vi "Obtain Broadcast Events.vi"(8 "error in (no error)":errorcluster, 10 "Create New? (F)":bool) -> (0 "error out":errorcluster, 2 "LV-WinSCP Broadcast Events":T1)   [LabVIEW 2015, in "LV-WinSCP.lvlib"]
doc: "This VI Obtains/Creates the Broadcast events that will be used for other modules to register to receive messages from the module that owns this VI.\n\n<b>NOTE</b>: The contents of this VI are automatically generated and modified by the <b>Tools > Delacor > DQMH</b> utilities. Consider using those utilities instead of making your own modifications to this VI.\n_____\nBased on DQMH Project Template 6.1.0.94."
uses:
  LV-WinSCP.lvlib
  Broadcast Events--cluster.ctl
  Did Init Argument--cluster.ctl
  Status Updated Argument--cluster.ctl
  Error Reported Argument--cluster.ctl
  Stop Argument--cluster.ctl
  Get Module Execution Status Argument--cluster.ctl
  Get Items From Target (Reply Payload)--cluster.ctl
  Classes/FileTransfer/FileAndDestination.ctl
  Classes/FileTransfer/TransferExceptionDescription.ctl
  Execute Command On Target (Reply Payload)--cluster.ctl
  Classes/CommandExecution/Status.ctl
  Classes/CommandExecution/ErrorDescription.ctl
  Send Items To Target (Reply Payload)--cluster.ctl
  Classes/FileTransfer/FileTransfer.lvclass
  Classes/CommandExecution/Command Execution.lvclass
panel:
  # "NOTE: The contents of this VI are automatically generated and modified by the Tools > Delacor > DQMH utilities. Consider using those utilities instead of making your own modifications to this VI."
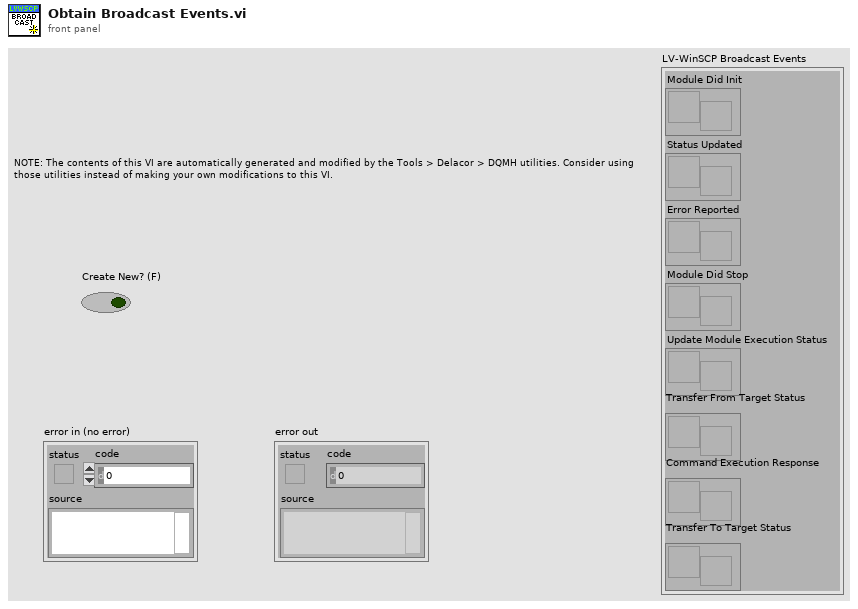
[diagram p1: front panel]
types:
  T1 = typedef "LV-WinSCP.lvlib/Broadcast Events--cluster.ctl" = cluster{"Module Did Init":refnum<user-event>, "Status Updated":refnum<user-event>, "Error Reported":refnum<user-event>, "Module Did Stop":refnum<user-event>, "Update Module Execution Status":refnum<user-event>, "Transfer From Target Status":refnum<user-event>, "Command Execution Response":refnum<user-event>, "Transfer To Target Status":refnum<user-event>}
  T2 = typedef "LV-WinSCP.lvlib/Send Items To Target (Reply Payload)--cluster.ctl" = cluster{"Transfer Succeeded":bool, "File Transfered Successfully":T3[], "Erroneous Transfers":T4[], "error":errorcluster}
  T3 = typedef "WinSCP.lvlib/FileTransfer.lvclass/FileAndDestination.ctl" = cluster{"FileName":string, "Destination":string}
  T4 = typedef "WinSCP.lvlib/FileTransfer.lvclass/TransferExceptionDescription.ctl" = cluster{"Message":string, "Source":string}
  T5 = typedef "LV-WinSCP.lvlib/Execute Command On Target (Reply Payload)--cluster.ctl" = cluster{"Status":T6, "Errors":T7[], "Sent Command":string, "error":errorcluster, "Output":string}
  T6 = typedef "WinSCP.lvlib/Command Execution.lvclass/Status.ctl" = cluster{"IsSuccess":bool, "ErrorOutput":string, "ExitCode":i32}
  T7 = typedef "WinSCP.lvlib/Command Execution.lvclass/ErrorDescription.ctl" = cluster{"Message":string, "Source":string}
  T8 = typedef "LV-WinSCP.lvlib/Get Items From Target (Reply Payload)--cluster.ctl" = cluster{"Transfer Succeeded":bool, "File Transfered Successfully":T3[], "Erroneous Transfers":T4[], "error":errorcluster}
  T9 = typedef "LV-WinSCP.lvlib/Get Module Execution Status Argument--cluster.ctl" = cluster{"Module ID":i32, "Running?":bool}
  T10 = typedef "LV-WinSCP.lvlib/Stop Argument--cluster.ctl" = cluster{"Module ID":i32, "Origin":string, "Exit via Stop Module Req?":bool, "Wait for Module to stop?":bool}
  T11 = typedef "LV-WinSCP.lvlib/Error Reported Argument--cluster.ctl" = cluster{"Error":errorcluster, "Additional Information":string, "Module ID":i32, "Module Name":string}
  T12 = typedef "LV-WinSCP.lvlib/Status Updated Argument--cluster.ctl" = cluster{"Status":string, "Module ID":i32}
  T13 = typedef "LV-WinSCP.lvlib/Did Init Argument--cluster.ctl" = cluster{"Init?":bool, "Info":string, "Module ID":i32}
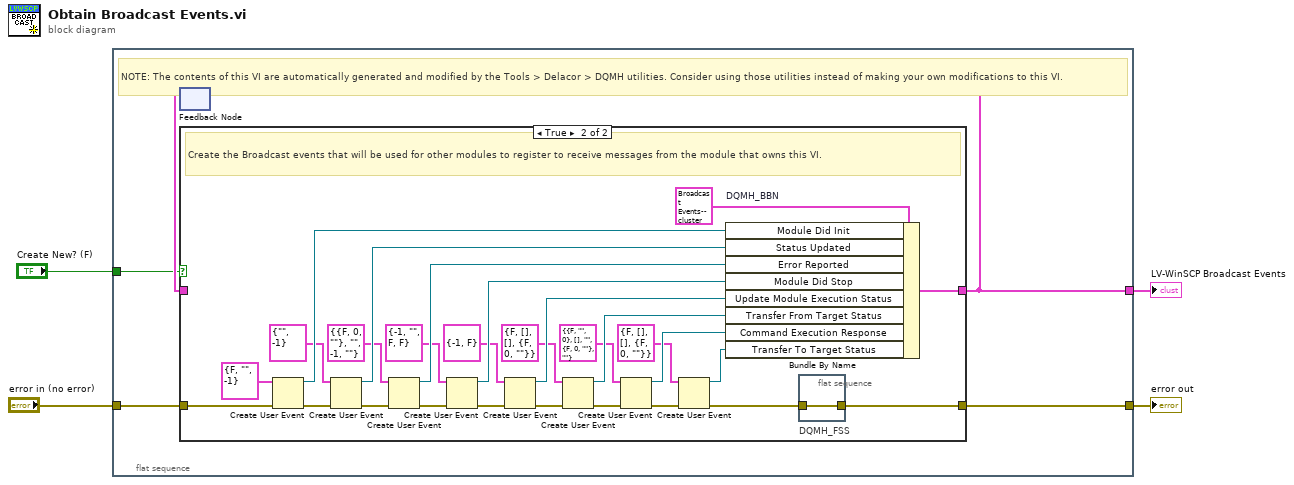
[diagram p0: block diagram]
diagram:
  n1 = flat-sequence {
    tunnel: [w9] -> w4
    tunnel: "error in (no error)" -> [w8]
    tunnel: [w6] -> w2
    tunnel: "Create New? (F)" -> [w5]
    frame #0 {
      # "NOTE: The contents of this VI are automatically generated and modified by the Tools > Delacor > DQMH utilities. Consider using those utilities instead of making your own modifications to this VI."
      n2 = feedback #1() -> (w7:T1)  [unwired: 1 in]
      n3 = case shown="True" w5 {
        tunnel: [w10 w24] -> w9
        tunnel: w8 -> [w10 w39]
        tunnel: [w11 w36] -> w6
        tunnel: w7 -> [w11 _]
        frame False {
          # "Obtain the Broadcast events that were created in a previous call to this VI."
        }
        frame True {
          # "Create the Broadcast events that will be used for other modules to register to receive messages from the module that owns this VI."
          n4 = Create User Event(user event datatype=T13 {"Init?"=FALSE, "Info"="", "Module ID"=-1} ("Did Init Argument"), error in=w39) -> (user event=w37:refnum<user-event>, error out=w34:errorcluster)
          n5 = Create User Event(user event datatype=T12 {"Status"="", "Module ID"=-1} ("Status Updated Argument"), error in=w34) -> (user event=w31:refnum<user-event>, error out=w33:errorcluster)
          n6 = Create User Event(user event datatype=T11 {"Error"={"status"=FALSE, "code"=0, "source"=""}, "Additional Information"="", "Module ID"=-1, "Module Name"=""} ("Error Reported Argument"), error in=w33) -> (user event=w28:refnum<user-event>, error out=w30:errorcluster)
          n7 = Create User Event(user event datatype=T10 {"Module ID"=-1, "Origin"="", "Exit via Stop Module Req?"=FALSE, "Wait for Module to stop?"=FALSE} ("Stop Argument"), error in=w30) -> (user event=w26:refnum<user-event>, error out=w25:errorcluster)
          n8 = Create User Event(user event datatype=T9 {"Module ID"=-1, "Running?"=FALSE} ("Get Module Execution Status Argument"), error in=w25) -> (user event=w22:refnum<user-event>, error out=w23:errorcluster)
          n9 = Create User Event(user event datatype=T8 {"Transfer Succeeded"=FALSE, "File Transfered Successfully"=[], "Erroneous Transfers"=[], "error"={"status"=FALSE, "code"=0, "source"=""}} ("Get Items From Target (Reply Payload)"), error in=w23) -> (user event=w19:refnum<user-event>, error out=w20:errorcluster)
          n10 = Create User Event(user event datatype=T5 {"Status"={"IsSuccess"=FALSE, "ErrorOutput"="", "ExitCode"=0}, "Errors"=[], "Sent Command"="", "error"={"status"=FALSE, "code"=0, "source"=""}, "Output"=""} ("Execute Command On Target (Reply Payload)"), error in=w20) -> (user event=w16:refnum<user-event>, error out=w17:errorcluster)
          n11 = Create User Event(user event datatype=T2 {"Transfer Succeeded"=FALSE, "File Transfered Successfully"=[], "Erroneous Transfers"=[], "error"={"status"=FALSE, "code"=0, "source"=""}} ("Send Items To Target (Reply Payload)"), error in=w17) -> (user event=w13:refnum<user-event>, error out=w14:errorcluster)
          n12 = Bundle By Name "DQMH_BBN"(cluster=T1 {"Module Did Init"=refnum, "Status Updated"=refnum, "Error Reported"=refnum, "Module Did Stop"=refnum, "Update Module Execution Status"=refnum, "Transfer From Target Status"=refnum, "Command Execution Response"=refnum, "Transfer To Target Status"=refnum} ("output cluster"), "Module Did Init"=w37, "Status Updated"=w31, "Error Reported"=w28, "Module Did Stop"=w26, "Update Module Execution Status"=w22, "Transfer From Target Status"=w19, "Command Execution Response"=w16, "Transfer To Target Status"=w13) -> (w36:T1)
          n13 = flat-sequence "DQMH_FSS" {
            tunnel: w14 -> [w40]
            tunnel: [w40] -> w24
            frame #0 {
            }
          }
        }
      }
      n14 = feedback-in #1(w6) -> ()
    }
  }
  "LV-WinSCP Broadcast Events" <- w2
  "error out" <- w4
